vi "sv_Fractional Octave Filtering (N Ch).vi"(0 "scaled signal(s) [EU]":waveform(dbl)[](array[waveform]), 1 "reset filter (F)":bool, 5 "1/n octave settings":T3, 7 "midband frequency setting":T1, 11 "error in (no error)":errorcluster) -> (4 "filtered signal(s) [EU]":waveform(dbl)[](array[waveform]), 6 "settled?":bool, 8 "actual midband frequency [Hz]":dbl, 15 "error out":errorcluster)   [LabVIEW 2017, in "SoundVib_Octave_2014 standard.lvlib"]
doc: "This VI designs a single octave filter based on the specified midband frequency and bandwidth and applies the filter to input time domain signal.\n\nThe fractional-octave filter is designed in accordance with one of the following standards:\n ANSI S1.11-2014;\n IEC 61260-1:2014.\nFor both standards, the sampling frequency must be at least 3 times the highest midband frequency for octave analysis and at least 2.5 times the highest midband frequency for 1/3, 1/6, 1/12, or 1/24 octave analysis. Available bandwidths are 1/1, 1/3, 1/6, 1/12, and 1/24 octave.\n\nTo ensure a continuous filtering operation, call this VI the first time with reset filter set to TRUE and then call it with reset filter set to FALSE.\n\nTo design a standard octave filter, set coerce to nearest standard midband frequency to TRUE."
uses:
  <vilib>/addons/Sound and Vibration/svt_Octave/SoundVib_Octave_2014 standard.lvlib
  <vilib>/addons/_NISVFA/_Shared subVIs/Controls/svc_Octave Standard.ctl
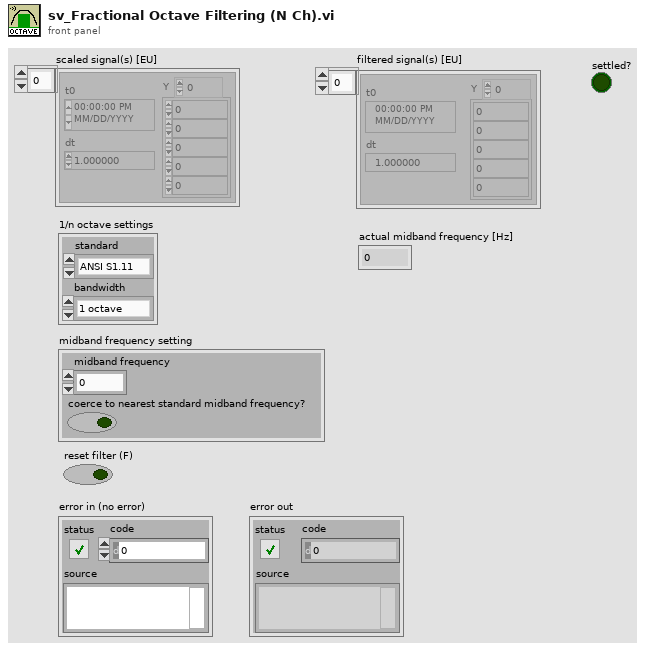
[diagram p1: front panel]
types:
  T1 = cluster{"midband frequency":dbl, "coerce to nearest standard midband frequency?":bool}
  T2 = typedef "svc_Octave Standard.ctl" = enum16{"ANSI S1.11", "IEC 61260"}
  T3 = cluster{"standard":T2, "bandwidth":enum16{"1 octave", "1/3 octave", "1/6 octave", "1/12 octave", "1/24 octave"}}
  T4 = enum16{"1 octave", "1/3 octave", "1/6 octave", "1/12 octave", "1/24 octave"}
  T5 = typedef "svc_Octave Filter Bank Parameters.ctl" = cluster{"octave filter coefficients":cluster{"filter structure":enum32{"IIR 2nd Order", "IIR 4th Order"}, "Reverse Coefficients":dbl[], "Forward Coefficients":dbl[]}[], "lowpass filter coefficients":cluster{"filter structure":enum32{"IIR 2nd Order", "IIR 4th Order"}, "Reverse Coefficients":dbl[], "Forward Coefficients":dbl[]}, "number of samples to settle":u64, "number of decimation steps required":i32[], "octave filter bandwidth":dbl[]}
  T6 = typedef "svc_Octave Filter State.ctl" = cluster{"octave filter":cluster{"Octave filter":dbl[]}[], "lowpass filter":dbl[][], "exponential averaging":cluster{"exponential averaging":dbl, "peak detector":dbl}[], "linear averaging":cluster{"squared sum":dbl, "size":dbl}[], "result":dbl[], "number of samples since init":u64, "decimation":dbl[]}
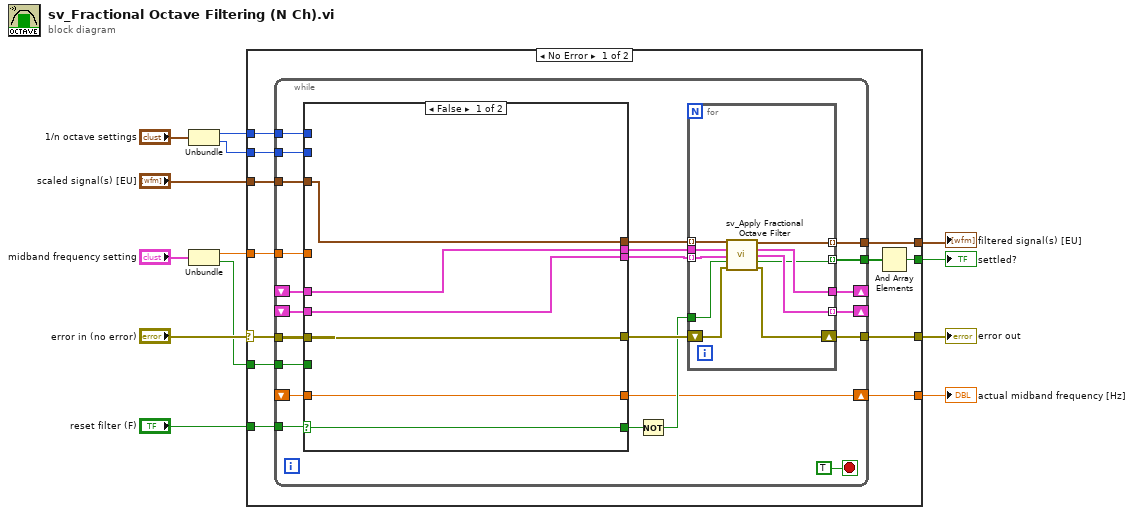
[diagram p0: block diagram]
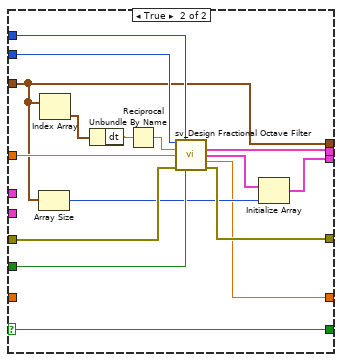
[diagram p2: hidden frame]
diagram:
  n1 = Unbundle("1/n octave settings") -> ("standard"=w6:T2, "bandwidth"=w5:T4)
  n2 = Unbundle("midband frequency setting") -> ("midband frequency"=w2:dbl, "coerce to nearest standard midband frequency?"=w3:bool)
  n3 = case shown="No Error" "error in (no error)" {
    selector: "error in (no error)" -> [w19 w81]
    tunnel: w2 -> [w25 _]
    tunnel: w3 -> [w24 _]
    tunnel: w5 -> [w23 _]
    tunnel: w6 -> [w22 _]
    tunnel: "scaled signal(s) [EU]" -> [w21 _]
    tunnel: [w17 w81] -> w13
    tunnel: "reset filter (F)" -> [w20 _]
    tunnel: [w18 _] -> w9
    tunnel: [w15 _] -> w8
    tunnel: [w14 _] -> w1
    frame No Error {
      n4 = while {
        tunnel: w25 -> [w48]
        tunnel: w24 -> [w47]
        tunnel: w23 -> [w46]
        tunnel: w22 -> [w45]
        tunnel: w20 -> [w41]
        tunnel: w19 -> [w43]
        tunnel: w21 -> [w44]
        shift-right: [w32] -> _
        shift-left: _ -> [w39]
        shift-right: [w33] -> _
        shift-left: _ -> [w38]
        tunnel: [w34] -> w18
        tunnel: [w31] -> w17
        tunnel: [w30] -> w16
        shift-right: [w27] -> w14
        shift-left: _ -> [w26]
        stop <- TRUE stop-if-true
        n5 = case shown="False" w41 {
          selector: w41 -> [w64 w74]
          tunnel: w48 -> [_ w80]
          tunnel: w47 -> [_ w79]
          tunnel: w46 -> [_ w78]
          tunnel: w45 -> [_ w77]
          tunnel: w44 -> [w60 w69]
          tunnel: w43 -> [w63 w76]
          tunnel: [w63 w75] -> w37
          tunnel: [w64 w74] -> w40
          tunnel: w39 -> [w61 _]
          tunnel: w38 -> [w62 _]
          tunnel: [w62 w66] -> w28
          tunnel: [w61 w72] -> w36
          tunnel: [w60 w69] -> w29
          tunnel: [w59 w65] -> w27
          tunnel: w26 -> [w59 _]
          frame False {
          }
          frame True {
            n6 = Array Size(array=w69) -> (size(s)=w67:i32)
            n7 = Index Array(array=w69) -> (element=w70:waveform(dbl))  [unwired: 1 in]
            n8 = Unbundle By Name(w70) -> ("dt"=w73:dbl)
            n9 = Reciprocal(x=w73) -> (1/x=w71:dbl)
            n10 = call <vilib>:"sv_Design Fractional Octave Filter.vi"("bandwidth"=w78, "standard"=w77, "sampling frequency [Hz]"=w71, "midband frequency [Hz]"=w80, "error in (no error)"=w76, "coerce to nearest standard midband frequency?"=w79) -> ("filter bank parameters"=w72:T5, "initial filter state"=w68:T6, "actual midband frequency [Hz]"=w65:dbl, "error out"=w75:errorcluster)  [unwired: 5 in, 1 out]
            n11 = Initialize Array(w68, w67) -> (w66:T6[])
          }
        }
        n12 = Not(x=w40) -> (.not. x?=w35:bool)
        n13 = for {
          tunnel: [w55] -> w34 mode=indexing
          tunnel: [w54] -> w33 mode=indexing
          shift-right: [w52] -> w31
          shift-left: w37 -> [w58]
          tunnel: w36 -> [w57]
          tunnel: [w53] -> w32
          tunnel: w35 -> [w56]
          tunnel: [w51] -> w30 mode=indexing
          tunnel: w29 -> [w50] mode=indexing
          tunnel: w28 -> [w49] mode=indexing
          n14 = call <vilib>:"sv_Apply Fractional Octave Filter.vi"("scaled signal [EU]"=w50, "filter bank parameters"=w57, "internal filter state IN"=w49, "filter init/cont (init:F)"=w56, "error in (no error)"=w58) -> ("filtered data"=w55:waveform(dbl), "dup filter bank parameters"=w53:T5, "internal filter state OUT"=w54:T6, "settled?"=w51:bool, "error out"=w52:errorcluster)  [unwired: 6 in]
        }
      }
      n15 = And Array Elements(Boolean array=w16) -> (logical AND=w15:bool)
    }
    frame Error {
    }
  }
  "error out" <- w13
  "filtered signal(s) [EU]" <- w9
  "settled?" <- w8
  "actual midband frequency [Hz]" <- w1
